vi "Main Tclk.vi"() -> ()   [LabVIEW 2018] (continued)
            n969 = property on="AF Steps" class="DigNum (strict)"("DisabledEnum"=w5460) -> ()  [unwired: 2 in, 2 out]
            n970 = property on="AS Steps" class="DigNum (strict)"("DisabledEnum"=w5460) -> ()  [unwired: 2 in, 2 out]
            n971 = property on="AA Steps" class="DigNum (strict)"("DisabledEnum"=w5460) -> ()  [unwired: 2 in, 2 out]
            n972 = property on="Beam blanked" class="Bool (strict)"("DisabledEnum"=w5460) -> ()  [unwired: 2 in, 2 out]
            n973 = property on="Spot" class="Bool (strict)"("DisabledEnum"=w5460) -> ()  [unwired: 2 in, 2 out]
            n974 = property on="Mill Stop" class="Bool (strict)"("DisabledEnum"=w5460) -> ()  [unwired: 2 in, 2 out]
            n975 = property on="ROI" class="Bool (strict)"("DisabledEnum"=w5460) -> ()  [unwired: 2 in, 2 out]
            n976 = property on="FIB Profile" class="Bool (strict)"("DisabledEnum"=w5460) -> ()  [unwired: 2 in, 2 out]
            n977 = property on="FIB FOV (um)" class="DigNum (strict)"("DisabledEnum"=w5460) -> ()  [unwired: 2 in, 2 out]
            n978 = property on="X center (um)" class="DigNum (strict)"("DisabledEnum"=w5460) -> ()  [unwired: 2 in, 2 out]
            n979 = property on="Z center (um)" class="DigNum (strict)"("DisabledEnum"=w5460) -> ()  [unwired: 2 in, 2 out]
            n980 = property on="X size (um)" class="DigNum (strict)"("DisabledEnum"=w5460) -> ()  [unwired: 2 in, 2 out]
            n981 = property on="Z size (um)" class="DigNum (strict)"("DisabledEnum"=w5460) -> ()  [unwired: 2 in, 2 out]
            n982 = property on="X resolution" class="DigNum (strict)"("DisabledEnum"=w5460) -> ()  [unwired: 2 in, 2 out]
            n983 = property on="Z resolution" class="DigNum (strict)"("DisabledEnum"=w5460) -> ()  [unwired: 2 in, 2 out]
            n984 = property on="Z-step (nm)" class="DigNum (strict)"("DisabledEnum"=w5460) -> ()  [unwired: 2 in, 2 out]
            n985 = property on="Start Current DataLog" class="Bool (strict)"("DisabledEnum"=w5460) -> ()  [unwired: 2 in, 2 out]
            n986 = local read "Machine Type"() -> (w5461:u8)
            n987 = local read "Unfreeze"() -> (w5468:bool)
            n988 = case shown="2" w5461 {
              frame 0, Default {
              }
              frame 2 {
                n989 = local read "Api"() -> (w5476:refnum<k7>)
                n990 = call "SmartSEM Remote API set float.vi"("vValue"=sgl 0.0, "lpszParam"="DP_PANEL_DISABLE", "Api"=w5476) -> ("Api out"=w5472:refnum<k7>)  [unwired: 7 in, 1 out]
                n991 = call "SmartSEM Remote API set float.vi"("vValue"=sgl 0.0, "lpszParam"="DP_JOYSTICK_DISABLE", "Api"=w5472) -> ()  [unwired: 7 in, 2 out]
              }
            }
            n992 = case shown="False" w5468 {
              tunnel: w5460 -> [w5477 _]
              frame False {
                n993 = property on="Pre image" class="Bool (strict)"("DisabledEnum"=w5477) -> ()  [unwired: 2 in, 2 out]
                n994 = property on="Post image" class="Bool (strict)"("DisabledEnum"=w5477) -> ()  [unwired: 2 in, 2 out]
                n995 = property on="Mill" class="Bool (strict)"("DisabledEnum"=w5477) -> ()  [unwired: 2 in, 2 out]
                n996 = property on="Mill Manual Pause" class="Bool (strict)"("DisabledEnum"=w5477) -> ()  [unwired: 2 in, 2 out]
              }
              frame True {
              }
            }
            n997 = property on="Pause for reheat" class="Bool (strict)"("DisabledEnum"=T44."Disabled and Grayed Out" ("Disabled")) -> ()  [unwired: 2 in, 2 out]
          }
          frame True {
            n998 = stacked-sequence {
              tunnel: [_ _ _ _ _ _ _ w5766 _ _ _ _ _ _ _ _ _ _ _ _ _ _ _ _ _ _ _ _ _ _ _ _ _ _ _ _ _ _ _ _ _ _ _] -> w5478
              frame #0 {
                w5479 = T44."Disabled and Grayed Out" ("Disabled")
                n999 = local read "FIB HW Config"() -> (w5490:T23)
                n1000 = local read "FIB HW Config"() -> (w5493:T23)
                n1001 = local read "Api"() -> (w5480:refnum<k7>)
                n1002 = Unbundle By Name(w5490) -> ("Beam blank"=w5491:tag)
                n1003 = Unbundle By Name(w5493) -> ("FIB Ext Scan"=w5494:tag)
                n1004 = local read "Milling para"() -> (w5486:T35)
                n1005 = property on="Pause for reheat" class="Bool (strict)"("DisabledEnum"=T44."Enabled" ("Disabled")) -> ()  [unwired: 2 in, 2 out]
                n1006 = property on="Scan x1" class="Bool (strict)"("DisabledEnum"=w5479) -> ()  [unwired: 2 in, 2 out]
                n1007 = property on="Mill start from Last" class="Bool (strict)"("DisabledEnum"=w5479) -> ()  [unwired: 2 in, 2 out]
                n1008 = property on="Scan xn" class="Bool (strict)"("DisabledEnum"=w5479) -> ()  [unwired: 2 in, 2 out]
                n1009 = property on="FIB Imaging" class="Bool (strict)"("DisabledEnum"=w5479) -> ()  [unwired: 2 in, 2 out]
                n1010 = property on="FIB time lapse" class="Bool (strict)"("DisabledEnum"=w5479) -> ()  [unwired: 2 in, 2 out]
                n1011 = property on="Reset" class="Bool (strict)"("DisabledEnum"=w5479) -> ()  [unwired: 2 in, 2 out]
                n1012 = property on="Pre image" class="Bool (strict)"("DisabledEnum"=w5479) -> ()  [unwired: 2 in, 2 out]
                n1013 = property on="Post image" class="Bool (strict)"("DisabledEnum"=w5479) -> ()  [unwired: 2 in, 2 out]
                n1014 = call "FIB ext scan.vi"("Ext on"=TRUE, "FIB Ext Scan"=w5494) -> ()  [unwired: 9 in, 1 out]
                n1015 = call "FIB beam blank.vi"("Api"=w5480, "Beam blanked"=TRUE, "lines"=w5491) -> ()  [unwired: 2 in, 1 out]
                n1016 = Unbundle By Name(w5486) -> ("Mill start from Last"=w5485:bool)
                n1017 = property on="Beam blanked" class="Bool (strict)"("DisabledEnum"=w5479) -> ()  [unwired: 2 in, 2 out]
                n1018 = property on="FIB Profile" class="Bool (strict)"("DisabledEnum"=w5479) -> ()  [unwired: 2 in, 2 out]
                n1019 = property on="Start Current DataLog" class="Bool (strict)"("DisabledEnum"=w5479) -> ()  [unwired: 2 in, 2 out]
                n1020 = property on="Spot" class="Bool (strict)"("DisabledEnum"=w5479) -> ()  [unwired: 2 in, 2 out]
                n1021 = property on="Mill Stop" class="Bool (strict)"("DisabledEnum"=w5479) -> ()  [unwired: 2 in, 2 out]
                n1022 = property on="ROI" class="Bool (strict)"("DisabledEnum"=w5479) -> ()  [unwired: 2 in, 2 out]
                n1023 = property on="Mill" class="Bool (strict)"("DisabledEnum"=w5479) -> ()  [unwired: 2 in, 2 out]
                n1024 = local read "FIB slice #"() -> (w5489:u32)
                n1025 = shared-variable "My Computer\\Zeiss Library.lvlib\\Milling cont. from Last"(w5485) -> ()  [unwired: 1 in, 1 out]
                n1026 = local write "SW error warning armed"(TRUE ("SW error warning armed")) -> ()
                n1027 = local write "Start Current DataLog"(FALSE ("Start Current DataLog")) -> ()
                n1028 = property on="FIB FOV (um)" class="DigNum (strict)"("DisabledEnum"=w5479) -> ()  [unwired: 2 in, 2 out]
                n1029 = property on="X center (um)" class="DigNum (strict)"("DisabledEnum"=w5479) -> ()  [unwired: 2 in, 2 out]
                n1030 = property on="X resolution" class="DigNum (strict)"("DisabledEnum"=w5479) -> ()  [unwired: 2 in, 2 out]
                n1031 = property on="Z resolution" class="DigNum (strict)"("DisabledEnum"=w5479) -> ()  [unwired: 2 in, 2 out]
                n1032 = property on="Z-step (nm)" class="DigNum (strict)"("DisabledEnum"=w5479) -> ()  [unwired: 2 in, 2 out]
                n1033 = property on="Z center (um)" class="DigNum (strict)"("DisabledEnum"=w5479) -> ()  [unwired: 2 in, 2 out]
                n1034 = property on="X size (um)" class="DigNum (strict)"("DisabledEnum"=w5479) -> ()  [unwired: 2 in, 2 out]
                n1035 = property on="Z size (um)" class="DigNum (strict)"("DisabledEnum"=w5479) -> ()  [unwired: 2 in, 2 out]
                n1036 = Equal To 0?(x=w5489) -> (x = 0?=w5488:bool)
                n1037 = And(x=w5488, y=w5485) -> (x .and. y?=w5487:bool)
                n1038 = case shown="True" w5487 {
                  frame False {
                  }
                  frame True {
                    n1039 = stacked-sequence {
                      frame #0 {
                        w5495 = TRUE ("Temperature warning armed")
                        n1040 = local read "Last FIB recipe"() -> (w5496:path)
                        n1041 = local write "Temperature warning armed"(w5495) -> ()
                        n1042 = local write "SW error warning armed"(w5495) -> ()
                        n1043 = local write "Focus index warning armed"(w5495) -> ()
                        n1044 = local write "Re-engage warning armed"(w5495) -> ()
                        n1045 = shared-variable ".\\Zeiss Library.lvlib\\FIB PID reset"(w5495) -> ()  [unwired: 1 in, 1 out]
                        n1046 = local write "Read recipe path"(w5496) -> ()
                      }
                      frame #1 {
                        n1047 = local write "Load recipe"(TRUE ("Load recipe")) -> ()
                      }
                      frame #2 {
                        n1048 = while {
                          stop <- w5498 stop-if-true
                          n1049 = local read "Load recipe"() -> (w5502:bool)
                          n1050 = Wait Until Next ms Multiple(millisecond multiple=u32 100) -> ()  [unwired: 1 out]
                          n1051 = local read "FIB"() -> (w5503:bool)
                          n1052 = local read "Stop"() -> (w5499:bool)
                          n1053 = Not(x=w5502) -> (.not. x?=w5501:bool)
                          n1054 = Not(x=w5503) -> (.not. x?=w5500:bool)
                          n1055 = Compound Arithmetic op=OR(w5501, w5500, w5499) -> (w5498:bool)
                        }
                      }
                      frame #3 {
                        n1056 = local read "Last milling snapshot"() -> (w5527:path)
                        n1057 = local read "Milling para"() -> (w5530:T35)
                        n1058 = local read "SEM Options"() -> (w5510:T27)
                        n1059 = local read "Last FIB image"() -> (w5539:path)
                        n1060 = local read "Last Det A Low Mag"() -> (w5537:path)
                        n1061 = local read "Last Det B Low Mag"() -> (w5538:path)
                        n1062 = shared-variable "My Computer\\Zeiss Library.lvlib\\Milling cont. from Last"(TRUE ("Milling cont. from Last")) -> ()  [unwired: 1 in, 1 out]
                        n1063 = local write "Initial Options"(w5510) -> ()
                        n1064 = local write "Reset Focus"(FALSE ("Reset Focus")) -> ()
                        n1065 = Bundle By Name(cluster=w5530, "Z offset (um)"=sgl 0.0 ("Y offset (um)")) -> (w5529:T35)
                        n1066 = call-poly <vilib>:"Read From XML File.vi"("XML File Path"=w5527) -> ("XML Elements"=w5526:string)  [unwired: 8 in, 2 out]
                        n1067 = File/Directory Info(path=w5539) -> (path out=w5541:path, error out=w5542:errorcluster)  [unwired: 1 in, 5 out]
                        n1068 = File/Directory Info(path=w5537) -> (path out=w5532:path, error out=w5531:errorcluster)  [unwired: 1 in, 5 out]
                        n1069 = File/Directory Info(path=w5538) -> (path out=w5535:path, error out=w5536:errorcluster)  [unwired: 1 in, 5 out]
                        n1070 = Unbundle By Name(w5542) -> ("status"=w5540:bool)
                        n1071 = Unbundle By Name(w5531) -> ("status"=w5533:bool)
                        n1072 = Unbundle By Name(w5536) -> ("status"=w5534:bool)
                        n1073 = local write "Milling para"(w5529) -> ()
                        n1074 = Unflatten From XML(xml string=w5526, type=T47 {"Timestamp"=timestamp(0 s since 1904-01-01), "Double"=0.0, "FIB slice #"=0, "Reheat"=FALSE, "Double 2"=0.0, "Double 3"=0.0, "Double 4"=0.0} ("output cluster")) -> (value=w5525:T47)  [unwired: 1 in, 1 out]
                        n1075 = case shown="False" w5540 {
                          tunnel: w5541 -> [w5558 _]
                          frame False {
                            n1076 = call <vilib>:"Read PNG File.vi"("path to PNG file"=w5558) -> ("image data"=w5559:T55)  [unwired: 8 in, 2 out]
                            n1077 = call <vilib>:"Unflatten Pixmap.vi"("image data"=w5559) -> ("8-bit pixmap"=w5557:u8[][])  [unwired: 4 in, 6 out]
                            n1078 = To Word Integer(number=w5557) -> (16bit integer=w5556:i16[][])
                            n1079 = local write "FIB Image"(w5556) -> ()
                            n1080 = shared-variable ".\\Zeiss Library.lvlib\\FIB Img"(w5556) -> ()  [unwired: 1 in, 1 out]
                          }
                          frame True {
                          }
                        }
                        n1081 = case shown="False" w5533 {
                          tunnel: w5532 -> [w5554 _]
                          frame False {
                            n1082 = call <vilib>:"Read PNG File.vi"("path to PNG file"=w5554) -> ("image data"=w5555:T55)  [unwired: 8 in, 2 out]
                            n1083 = call <vilib>:"Unflatten Pixmap.vi"("image data"=w5555) -> ("8-bit pixmap"=w5552:u8[][])  [unwired: 4 in, 6 out]
                            n1084 = To Word Integer(number=w5552) -> (16bit integer=w5553:i16[][])
                            n1085 = local write "Detector A Low Mag"(w5553) -> ()
                          }
                          frame True {
                          }
                        }
                        n1086 = case shown="False" w5534 {
                          tunnel: w5535 -> [w5550 _]
                          frame False {
                            n1087 = call <vilib>:"Read PNG File.vi"("path to PNG file"=w5550) -> ("image data"=w5551:T55)  [unwired: 8 in, 2 out]
                            n1088 = call <vilib>:"Unflatten Pixmap.vi"("image data"=w5551) -> ("8-bit pixmap"=w5549:u8[][])  [unwired: 4 in, 6 out]
                            n1089 = To Word Integer(number=w5549) -> (16bit integer=w5548:i16[][])
                            n1090 = local write "Detector B Low Mag"(w5548) -> ()
                          }
                          frame True {
                          }
                        }
                        n1091 = Unbundle(w5525) -> ("Timestamp"=w5522:timestamp, "Double"=w5524:sgl, "FIB slice #"=w5523:u32, "Reheat"=w5520:bool, "Double 2"=w5519:sgl, "Double 4"=w5506:sgl)  [unwired: 1 out]
                        "Reheat from last" <- w5520
                        n1092 = local read "Hardware Configuration"() -> (w5507:T25)
                        n1093 = Bundle By Name(cluster=w5507, "SEM Max FOV (um)"=w5506) -> (w5505:T25)
                        n1094 = Increment(x=w5523) -> (x+1=w5511:u32)
                        n1095 = case shown="True" w5520 {
                          tunnel: w5522 -> [_ w5547]
                          tunnel: w5519 -> [_ w5546]
                          frame False {
                            n1096 = local write "Pause for reheat"(FALSE ("Reheat")) -> ()
                            n1097 = property on="Pause for reheat" class="Bool (strict)"("DisabledEnum"=T44."Enabled" ("Disabled")) -> ()  [unwired: 2 in, 2 out]
                          }
                          frame True {
                            n1098 = local write "Pre-reheat time"(w5547) -> ()
                            n1099 = local write "Pre-reheat FI"(w5546) -> ()
                            n1100 = property on="Pause for reheat" class="Bool (strict)"("DisabledEnum"=T44."Disabled and Grayed Out" ("Disabled")) -> ()  [unwired: 2 in, 2 out]
                          }
                        }
                        n1101 = shared-variable ".\\Zeiss Library.lvlib\\Milling Z Voltage Last"(w5524) -> ()  [unwired: 1 in, 1 out]
                        n1102 = local write "FIB slice #"(w5511) -> ()
                        n1103 = local read "Email Alert Recipients"() -> (w5515:string[])
                        n1104 = local write "Hardware Configuration"(w5505) -> ()
                        n1105 = local read "Email recipents file"() -> (w5512:path)
                        n1106 = Open/Create/Replace File(file path (use dialog)=w5512, operation (0:open)=T49."replace or create") -> (refnum out=w5513:refnum<file>, error out=w5514:errorcluster)  [unwired: 4 in, 1 out]
                        n1107 = Write to Text File(file (use dialog)=w5513, text=w5515, error in=w5514) -> (refnum out=w5516:refnum<file>, error out=w5517:errorcluster)  [unwired: 1 in, 1 out]
                        n1108 = Close File(refnum=w5516, error in=w5517) -> ()  [unwired: 2 out]
                      }
                      frame #4 {
                        n1109 = local read "Reheat from last"() -> (w5560:bool)
                        n1110 = case shown="True" w5560 {
                          frame False {
                          }
                          frame True {
                            n1111 = local read "SEM Scan Parameters"() -> (w5565:T26)
                            n1112 = Unbundle By Name(w5565) -> ("X center (um)"=w5564:sgl, "Y center (um)"=w5563:sgl, "Y stig"=w5562:sgl[][])
                            n1113 = local write "Pre-reheat X center (um)"(w5564) -> ()
                            n1114 = local write "Pre-reheat Y center (um)"(w5563) -> ()
                            n1115 = local write "Pre-reheat Y stig"(w5562) -> ()
                            n1116 = local write "Status Tabs"(T11."Re-engage" ("Status Tabs")) -> ()
                          }
                        }
                      }
                    }
                  }
                }
              }
              frame #1 {
                n1117 = local read "Machine Type"() -> (w5582:u8)
                n1118 = local read "Milling para"() -> (w5580:T35)
                n1119 = Unbundle By Name(w5580) -> ("Lines auto pause"=w5579:u16)
                n1120 = case shown="2" w5582 {
                  tunnel: [w5591 w5599 w5603] -> w5583
                  frame 0, Default {
                    n1121 = for {
                      N: 10 -> [_]
                      tunnel: [w5596] -> w5593 mode=indexing
                      n1122 = shared-variable ".\\Zeiss Library.lvlib\\Logs"() -> (w5598:sgl[])  [unwired: 1 in, 1 out]
                      n1123 = Wait Until Next ms Multiple(millisecond multiple=u32 10) -> ()  [unwired: 1 out]
                      n1124 = Index Array(array=w5598, index=0) -> (element=w5596:sgl)
                    }
                    n1125 = call-poly <vilib>:"Basic Averaged DC-RMS.vi"("signal in"=w5593) -> ("DC value"=w5592:dbl)  [unwired: 7 in, 3 out]
                    n1126 = To Single Precision Float(number=w5592) -> (single precision float=w5591:sgl)
                  }
                  frame 1 {
                    n1127 = local read "Faraday Cup (nA)"() -> (w5599:sgl)
                  }
                  frame 2 {
                    n1128 = local read "Api"() -> (w5602:refnum<k7>)
                    n1129 = for {
                      N: 10 -> [_]
                      tunnel: [w5608] -> w5605 mode=indexing
                      n1130 = shared-variable ".\\Zeiss Library.lvlib\\Logs"() -> (w5610:sgl[])  [unwired: 1 in, 1 out]
                      n1131 = Wait Until Next ms Multiple(millisecond multiple=u32 10) -> ()  [unwired: 1 out]
                      n1132 = Index Array(array=w5610, index=0) -> (element=w5608:sgl)
                    }
                    n1133 = call "SmartSEM Remote API set float.vi"("vValue"=sgl 1.0, "lpszParam"="DP_PANEL_DISABLE", "Api"=w5602) -> ()  [unwired: 7 in, 2 out]
                    n1134 = call-poly <vilib>:"Basic Averaged DC-RMS.vi"("signal in"=w5605) -> ("DC value"=w5604:dbl)  [unwired: 7 in, 3 out]
                    n1135 = To Single Precision Float(number=w5604) -> (single precision float=w5603:sgl)
                  }
                }
                "Faraday Cup before mill" <- w5583
                n1136 = Equal?(x=w5579, y=u16 1) -> (x = y?=w5572:bool)
                n1137 = case shown="True" w5572 {
                  tunnel: [0 w5585] -> w5571
                  frame False {
                  }
                  frame True {
                    n1138 = local read "Continued fine milling frames"() -> (w5586:i32)
                    n1139 = Increment(x=w5586) -> (x+1=w5585:i32)
                  }
                }
                n1140 = local read "EHT off"() -> (w5575:bool)
                n1141 = local read "Faraday Cup (nA)"() -> (w5577:sgl)
                n1142 = local read "SEM Options"() -> (w5581:T27)
                n1143 = Not(x=w5575) -> (.not. x?=w5574:bool)
                n1144 = Unbundle By Name(w5581) -> ("Upload"=w5567:bool)
                n1145 = Greater?(x=w5577, y=sgl 0.1) -> (0:w5573:bool)
                n1146 = shared-variable ".\\Zeiss Library.lvlib\\Faraday Cup before mill"(w5583) -> ()  [unwired: 1 in, 1 out]
                n1147 = local write "Continued fine milling frames"(w5571) -> ()
                n1148 = Greater?(x=w5571, y=5) -> (0:w5569:bool)
                n1149 = Compound Arithmetic op=AND(w5569, w5574, w5573) -> (w5568:bool)
                n1150 = Or(x=w5568, y=w5567) -> (x .or. y?=w5566:bool)
                n1151 = case shown="True" w5566 {
                  frame False {
                  }
                  frame True {
                    w5588 = TRUE ("Upload")
                    n1152 = local read "Alert Settings"() -> (w5590:T36)
                    n1153 = Bundle By Name(cluster=w5590, "3D imaging paused alarm"=w5588, "FIB emission warning"=w5588, "Specimen @ SEM alarm"=w5588, "FIB CL current alarm"=w5588, "Beam Dump 1 alarm"=w5588, "Milling Z voltage alarm"=w5588, "EHT off alarm"=w5588, "Image clipping alarm"=w5588, "Temperature alarm"=w5588, "SW error warning"=w5588, "Focus index warning"=w5588) -> (w5589:T36)
                    n1154 = local write "Coarse milling"(FALSE ("Coarse milling")) -> ()
                    n1155 = local write "Alert Settings"(w5589) -> ()
                  }
                }
              }
              frame #2 {
                w5612 = FALSE ("Rect Milling Line Paused")
                w5613 = TRUE ("Auto pause")
                n1156 = local read "Milling para"() -> (w5611:T35)
                n1157 = Bundle By Name(cluster=w5611, "Auto pause"=w5613) -> (w5614:T35)
                n1158 = shared-variable "My Computer\\Zeiss Library.lvlib\\Milling Resume"(w5613) -> ()  [unwired: 1 in, 1 out]
                n1159 = shared-variable "My Computer\\Zeiss Library.lvlib\\Milling Line Paused"(w5612) -> ()  [unwired: 1 in, 1 out]
                n1160 = local write "Mill Stop"(w5612) -> ()
                n1161 = local write "Milling para"(w5614) -> ()
              }
              frame #3 {
                n1162 = local read "FIB slice #"() -> (w5616:u32)
                n1163 = Equal To 0?(x=w5616) -> (x = 0?=w5615:bool)
                n1164 = case shown="True" w5615 {
                  frame False {
                  }
                  frame True {
                    n1165 = stacked-sequence {
                      frame #0 {
                        w5630 = 0.0
                        w5641 = TRUE ("Temperature warning armed")
                        w5619 = u32[] [] ("Log time array")
                        w5617 = sgl[] []
                        n1166 = local write "SW error warning armed"(w5641) -> ()
                        n1167 = local write "Focus index warning armed"(w5641) -> ()
                        n1168 = local write "Temperature warning armed"(w5641) -> ()
                        n1169 = local write "Re-engage warning armed"(w5641) -> ()
                        n1170 = shared-variable ".\\Zeiss Library.lvlib\\FIB PID reset"(w5641) -> ()  [unwired: 1 in, 1 out]
                        n1171 = Get Date/Time In Seconds() -> (seconds since 1Jan1904=w5640:timestamp)
                        n1172 = To Double Precision Float(number=w5640) -> (double precision float=w5635:dbl)
                        n1173 = Bundle(w5630, w5630) -> (w5629:cluster{dbl, dbl})  [unwired: 1 in]
                        n1174 = Add(x=w5635, y=86400.0 ("X Scale.Range:Maximum")) -> (x+y=w5637:dbl)
                        n1175 = Initialize Array(w5629, 0) -> (w5632:cluster{dbl, dbl}[])
                        n1176 = Add(x=w5635, y=0.0 ("X Scale.Range:Minimum")) -> (x+y=w5633:dbl)
                        n1177 = local read "SEM Scan Parameters"() -> (w5623:T26)
                        n1178 = property on="FIB HV DataLog" class="WFChart (strict)"("History Data"=w5632, "XScale.Offset"=w5635, "XScale.Minimum"=w5633, "XScale.Maximum"=w5637, "XScale.Increment"=14400.0 ("X Scale.Range:Increment"), "XScale.MinorInc"=3600.0 ("X Scale.Range:Minor Increment")) -> ()  [unwired: 2 in, 2 out]
                        n1179 = Unbundle By Name(w5623) -> ("Y tiles"=w5622:u8, "X tiles"=w5621:u8)
                        n1180 = Initialize Array(FALSE ("run minimized? (F)"), w5622, w5621) -> (w5624:bool[][])
                        n1181 = local read "3D FIB-SEM Files"() -> (w5627:path)
                        n1182 = local write "AF Success tiled"(w5624) -> ()
                        n1183 = local write "ASX Success tiled"(w5624) -> ()
                        n1184 = local write "ASY Success tiled"(w5624) -> ()
                        n1185 = local write "AAX Success tiled"(w5624) -> ()
                        n1186 = local write "AAY Success tiled"(w5624) -> ()
                        n1187 = local write "Auto re-engage"(FALSE ("Auto re-engage")) -> ()
                        n1188 = call <vilib>:"System Exec.vi"("run minimized? (F)"=TRUE, "working directory"=w5627, "command line"="cmd /c del Primary_grid*.png pre*.png post*.png") -> ()  [unwired: 5 in, 4 out]
                        "Temp array" <- w5617
                        "Faraday Cup array" <- w5617
                        "Specimen I array" <- w5617
                        "Beam Dump 1 array" <- w5617
                        "Log time array" <- w5619
                        "Delta X array" <- w5617
                        "Delta Y array" <- w5617
                        "Delta image array" <- w5617
                        "Focus index array" <- w5617
                        "Delta X sum array" <- w5617
                        "Delta Y sum array" <- w5617
                        "SEM Specimen I array" <- w5617
                        "Milling Z voltage array" <- w5617
                        "Delta Z array" <- w5617
                        "Beam Dump 2 array" <- w5617
                        "Milling I array" <- w5617
                        "Temp low limit array" <- w5617
                        "Temp high limit array" <- w5617
                        "SEM Specimen I low limit array" <- w5617
                        "SEM Specimen I high limit array" <- w5617
                        "FI low limit array" <- w5617
                        "Specimen I low limit array" <- w5617
                        "Specimen I high limit array" <- w5617
                        "Faraday Cup low limit array" <- w5617
                        "Faraday Cup high limit array" <- w5617
                        "Cycle time array" <- w5619
                        "Cycle time est offset array" <- i16[] [] ("Log time array")
                        "BD1 low limit array" <- w5617
                        "BD1 high limit array" <- w5617
                        "BD2 low limit array" <- w5617
                        "BD2 high limit array" <- w5617
                        "Milling I low limit array" <- w5617
                        "Milling I high limit array" <- w5617
                        "FI low warning limit array" <- w5617
                        "FI high warning limit array" <- w5617
                        "FI low stop limit array" <- w5617
                        "FI high stop limit array" <- w5617
                        "Delta X stop limit array" <- w5617
                        "Delta Y stop limit array" <- w5617
                        "FI array for stop limit" <- w5617
                        "Delta X array for stop limit" <- w5617
                        "Delta Y array for stop limit" <- w5617
                      }
                      frame #1 {
                        n1189 = local read "SEM Scan Parameters"() -> (w5668:T26)
                        n1190 = Unbundle By Name(w5668) -> ("WD (mm)"=w5667:sgl[][], "X stig"=w5664:sgl[][], "Y stig"=w5661:sgl[][], "X aln"=w5660:sgl[][], "Y aln"=w5658:sgl[][], "dX (um)"=w5656:sgl[], "dY (um)"=w5651:sgl[], "Y tiles"=w5654:u8, "X tiles"=w5652:u8)
                        n1191 = local read "WD Stig Aln tile offsets"() -> (w5670:T3)
                        n1192 = Build Array(w5654, w5652) -> (w5657:u8[])
                        n1193 = Array Size(array=w5667) -> (size(s)=w5666:i32[])
                        n1194 = Array Size(array=w5664) -> (size(s)=w5665:i32[])
                        n1195 = Array Size(array=w5661) -> (size(s)=w5662:i32[])
                        n1196 = Array Size(array=w5660) -> (size(s)=w5663:i32[])
                        n1197 = Array Size(array=w5658) -> (size(s)=w5659:i32[])
                        n1198 = Array Size(array=w5656) -> (size(s)=w5655:i32)
                        n1199 = Array Size(array=w5651) -> (size(s)=w5653:i32)
                        n1200 = Equal?(x=w5666, y=w5657) -> (x = y?=w5649:bool[])
                        n1201 = Equal?(x=w5665, y=w5657) -> (x = y?=w5648:bool[])
                        n1202 = Equal?(x=w5662, y=w5657) -> (x = y?=w5646:bool[])
                        n1203 = Equal?(x=w5663, y=w5657) -> (x = y?=w5645:bool[])
                        n1204 = Equal?(x=w5659, y=w5657) -> (x = y?=w5644:bool[])
                        n1205 = Equal?(x=w5655, y=w5654) -> (x = y?=w5643:bool)
                        n1206 = Equal?(x=w5653, y=w5652) -> (x = y?=w5642:bool)
                        n1207 = Build Array (concatenate)(w5649, w5648, w5646, w5645, w5644, w5643, w5642) -> (w5647:bool[])
                        n1208 = And Array Elements(Boolean array=w5647) -> (logical AND=w5650:bool)
                        n1209 = case shown="True" w5650 {
                          tunnel: [w5671 w5699] -> w5669
                          tunnel: w5668 -> [w5673 w5693]
                          tunnel: w5670 -> [w5672 w5680]
                          frame False {
                            w5675 = sgl 0.0 ("element")
                            n1210 = Unbundle By Name(w5673) -> ("Y tiles"=w5677:u8, "X tiles"=w5679:u8)
                            n1211 = Initialize Array(w5675, w5677, w5679) -> (w5678:sgl[][])
                            n1212 = Initialize Array(w5675, w5677) -> (w5676:sgl[])
                            n1213 = Initialize Array(w5675, w5679) -> (w5674:sgl[])
                            n1214 = Bundle By Name(cluster=w5672, "dWD"=w5678, "dX stig"=w5678, "dY stig"=w5678, "dX aln"=w5678, "dY aln"=w5678, "dX (um)"=w5676, "dY (um)"=w5674) -> (w5671:T3)
                          }
                          frame True {
                            n1215 = Unbundle By Name(w5693) -> ("WD (mm)"=w5689:sgl[][], "X stig"=w5687:sgl[][], "Y stig"=w5684:sgl[][], "X aln"=w5683:sgl[][], "Y aln"=w5681:sgl[][], "dX (um)"=w5700:sgl[], "dY (um)"=w5705:sgl[], "Y tiles"=w5692:u8, "X tiles"=w5691:u8)
                            n1216 = expression code="(x-1)/2"(w5692) -> (w5703:u8)
                            n1217 = expression code="(x-1)/2"(w5691) -> (w5706:u8)
                            n1218 = Index Array(array=w5689, index (row)=w5703, index (col)=w5706) -> (element=w5690:sgl)
                            n1219 = Index Array(array=w5687, index (row)=w5703, index (col)=w5706) -> (element=w5688:sgl)
                            n1220 = Index Array(array=w5684, index (row)=w5703, index (col)=w5706) -> (element=w5685:sgl)
                            n1221 = Index Array(array=w5683, index (row)=w5703, index (col)=w5706) -> (element=w5686:sgl)
                            n1222 = Index Array(array=w5681, index (row)=w5703, index (col)=w5706) -> (element=w5682:sgl)
                            n1223 = Index Array(array=w5700, index=w5703) -> (element=w5701:sgl)
                            n1224 = Index Array(array=w5705, index=w5706) -> (element=w5704:sgl)
                            n1225 = Subtract(x=w5689, y=w5690) -> (x-y=w5694:sgl[][])
                            n1226 = Subtract(x=w5687, y=w5688) -> (x-y=w5695:sgl[][])
                            n1227 = Subtract(x=w5684, y=w5685) -> (x-y=w5696:sgl[][])
                            n1228 = Subtract(x=w5683, y=w5686) -> (x-y=w5697:sgl[][])
                            n1229 = Subtract(x=w5681, y=w5682) -> (x-y=w5698:sgl[][])
                            n1230 = Subtract(x=w5700, y=w5701) -> (x-y=w5702:sgl[])
                            n1231 = Subtract(x=w5705, y=w5704) -> (x-y=w5707:sgl[])
                            n1232 = Bundle By Name(cluster=w5680, "dWD"=w5694, "dX stig"=w5695, "dY stig"=w5696, "dX aln"=w5697, "dY aln"=w5698, "dX (um)"=w5702, "dY (um)"=w5707) -> (w5699:T3)
                          }
                        }
                        n1233 = local write "WD Stig Aln tile offsets"(w5669) -> ()
                      }
                    }
                  }
                }
              }
              frame #4 {
                n1234 = Unbundle By Name("Low Mag SEM") -> ("Low mag scan"=w5710:bool)
                n1235 = Unbundle By Name("Mid Mag SEM") -> ("Mid mag scan"=w5711:bool)
                n1236 = case shown="True" w5710 {
                  tunnel: "Low Mag SEM" -> [_ w5734]
                  frame False {
                  }
                  frame True {
                    w5730 = sgl[] [0.0] ("dX (um)")
                    w5731 = u8 1 ("X tiles")
                    w5735 = 0.0 ("X center")
                    n1237 = Unbundle By Name(w5734) -> ("Low mag scan FOV (micron)"=w5732:dbl, "Low mag scan rate (Hz)"=w5744:u32)
                    n1238 = local read "SEM Scan Parameters"() -> (w5737:T26)
                    n1239 = Unbundle By Name(w5737) -> ("Scan rate (Hz)"=w5739:u32, "Oversampling"=w5738:u32)
                    n1240 = expression code="x*1000"(w5732) -> (w5745:dbl)
                    n1241 = Multiply(x=w5739, y=w5738) -> (x*y=w5740:u32)
                    n1242 = Divide(x=w5740, y=w5744) -> (x/y=w5741:dbl)
                    n1243 = Divide(x=w5745, y=u32 512 ("X resolution")) -> (x/y=w5743:dbl)
                    n1244 = Bundle By Name(cluster=w5737, "X size (um)"=w5732, "Y size (um)"=w5732, "X center (um)"=w5735, "Y center (um)"=w5735, "X size (V)"=20.0, "Scan rate (Hz)"=w5744, "Oversampling"=w5741, "X tiles"=w5731, "Y tiles"=w5731, "Frames"=w5731, "dX (um)"=w5730, "dY (um)"=w5730, "Pixel size (nm)"=w5743) -> (→"SEM Low Mag Scan Parameters":T26)
                  }
                }
                n1245 = case shown="True" w5711 {
                  tunnel: "Mid Mag SEM" -> [_ w5718]
                  frame False {
                  }
                  frame True {
                    w5712 = sgl[] [0.0] ("dX (um)")
                    w5713 = u8 1 ("X tiles")
                    n1246 = local read "SEM Scan Parameters"() -> (w5719:T26)
                    n1247 = Unbundle By Name(w5718) -> ("X size (um)"=w5725:sgl, "Y size (um)"=w5726:sgl, "X center (um)"=w5727:dbl, "Y center (um)"=w5728:dbl, "Mid mag scan rate (Hz)"=w5724:u32, "Pixel size (nm)"=w5729:sgl)
                    n1248 = local read "SEM Mid Mag Scan Parameters"() -> (w5716:T5)
                    n1249 = Unbundle By Name(w5719) -> ("Scan rate (Hz)"=w5721:u32, "Oversampling"=w5720:u32)
                    n1250 = Unbundle By Name(w5716) -> ("X size (V)"=w5715:dbl)
                    n1251 = Multiply(x=w5721, y=w5720) -> (x*y=w5722:u32)
                    n1252 = Divide(x=w5722, y=w5724) -> (x/y=w5723:dbl)
                    n1253 = Bundle By Name(cluster=w5719, "X size (um)"=w5725, "Y size (um)"=w5726, "X center (um)"=w5727, "Y center (um)"=w5728, "Oversampling auto"=TRUE ("X size auto"), "Scan rate (Hz)"=w5724, "Oversampling"=w5723, "Pixel size (nm)"=w5729, "X size (V)"=w5715, "X tiles"=w5713, "Y tiles"=w5713, "Frames"=w5713, "dX (um)"=w5712, "dY (um)"=w5712) -> (→"SEM Mid Mag Scan Parameters":T26)
                  }
                }
              }
              frame #5 {
                w5746 = TRUE ("Mill")
                n1254 = local write "Mill"(w5746) -> ()
                n1255 = local write "Run once"(w5746) -> ()
                n1256 = Wait (ms)(milliseconds to wait=u32 200) -> ()  [unwired: 1 out]
              }
              frame #6 {
                n1257 = shared-variable ".\\Zeiss Library.lvlib\\Milling Z Voltage"() -> (w5749:sgl)  [unwired: 1 in, 1 out]
                n1258 = local read "FIB Options"() -> (w5758:T33)
                n1259 = local read "FIB Scan Parameters"() -> (w5756:T32)
                n1260 = local read "Milling para"() -> (w5755:T35)
                n1261 = Unbundle By Name(w5758) -> ("Flip z"=w5763:bool)
                n1262 = Unbundle By Name(w5755) -> ("FIB FOV (um)"=w5762:sgl)
                n1263 = Unbundle By Name(w5755) -> ("X size (um)"=w5753:sgl, "Line milling time (s)"=w5751:sgl, "Lines auto pause"=w5750:u16)
                n1264 = Unbundle By Name(w5756) -> ("Z size (V)"=w5757:dbl)
                n1265 = Negate(x=w5749) -> (-x=w5759:sgl)
                n1266 = Select(t=w5759, s=w5763, f=w5749) -> (s? t:f=w5760:sgl)
                n1267 = Divide(x=w5760, y=w5757) -> (x/y=w5761:dbl)
                n1268 = Multiply(x=w5761, y=w5762) -> (x*y=w5748:dbl)
                n1269 = call "Milling parameter to trapezoidal shape.vi"("Y location (um)"=w5748, "Milling para"=w5755) -> ("X size (um) @ Y"=w5754:dbl)  [unwired: 5 in, 4 out]
                n1270 = Divide(x=w5754, y=w5753) -> (x/y=w5752:dbl)
                n1271 = Compound Arithmetic op=MULTIPLY(w5752, w5751, w5750) -> (w5764:dbl)
                n1272 = local write "Milling time (s)"(w5764) -> ()
              }
              frame #7 {
                n1273 = while {
                  tunnel: [w5795] -> w5766
                  tunnel: [w5789] -> w5767
                  i -> [w5771]
                  stop <- w5796 stop-if-true
                  n1274 = Get Date/Time In Seconds() -> (seconds since 1Jan1904=w5785:timestamp)
                  n1275 = local read "Re-engage time"() -> (w5779:timestamp)
                  n1276 = local read "Milling para"() -> (w5782:T35)
                  n1277 = local read "Pre-reheat FIB PID target"() -> (w5778:sgl)
                  n1278 = local read "Run once"() -> (w5776:bool)
                  n1279 = shared-variable "My Computer\\Zeiss Library.lvlib\\Milling Line Paused"() -> (w5790:bool)  [unwired: 1 in, 1 out]
                  n1280 = local read "Mill Manual Pause"() -> (w5794:bool)
                  n1281 = local read "Machine Type"() -> (w5772:u8)
                  n1282 = local read "Auto reheat running"() -> (w5770:bool)
                  n1283 = local read "Reheat Output"() -> (w5788:T21)
                  n1284 = local read "Stop"() -> (w5795:bool)
                  n1285 = Wait Until Next ms Multiple(millisecond multiple=u32 100 ("milliseconds to wait")) -> ()  [unwired: 1 out]
                  n1286 = Unbundle By Name(w5782) -> ("FIB PID on"=w5780:bool)
                  n1287 = local read "FIB"() -> (w5792:bool)
                  n1288 = Subtract(x=w5785, y=w5779) -> (x-y=w5784:dbl)
                  n1289 = Unbundle By Name(w5788) -> ("Reheat Success"=w5787:bool)
                  n1290 = Not Equal To 0?(x=w5778) -> (x != 0?=w5775:bool)
                  n1291 = Not(x=w5792) -> (.not. x?=w5789:bool)
                  n1292 = expression code="x/60"(w5784) -> (w5777:dbl)
                  n1293 = case shown="True" w5794 {
                    tunnel: T44."Disabled and Grayed Out" ("Disabled") -> [w5891 _]
                    tunnel: T44."Enabled" ("Disabled") -> [_ w5909]
                    tunnel: w5772 -> [w5890 w5908]
                    tunnel: w5771 -> [w5889 w5907]
                    tunnel: w5770 -> [_ w5906]
                    frame False {
                      n1294 = stacked-sequence {
                        tunnel: w5891 -> [_ w5896 w5897 _ _]
                        tunnel: w5890 -> [_ _ _ w5898 w5902]
                        tunnel: w5889 -> [w5893 _ _ _ _]
                        frame #0 {
                          n1295 = Equal To 0?(x=w5893) -> (x = 0?=w5892:bool)
                          n1296 = case shown="True" w5892 {
                            frame False {
                            }
                            frame True {
                              n1297 = local write "Start Current DataLog"(FALSE ("Start Current DataLog")) -> ()
                              n1298 = local write "Status message"("FIB milling ..." ("Status message")) -> ()
                            }
                          }
                        }
                        frame #1 {
                          n1299 = property on="Scan x1" class="Bool (strict)"("DisabledEnum"=w5896) -> ()  [unwired: 2 in, 2 out]
                          n1300 = property on="Scan xn" class="Bool (strict)"("DisabledEnum"=w5896) -> ()  [unwired: 2 in, 2 out]
                          n1301 = property on="Pre image" class="Bool (strict)"("DisabledEnum"=w5896) -> ()  [unwired: 2 in, 2 out]
                          n1302 = property on="Post image" class="Bool (strict)"("DisabledEnum"=w5896) -> ()  [unwired: 2 in, 2 out]
                          n1303 = property on="Reset" class="Bool (strict)"("DisabledEnum"=w5896) -> ()  [unwired: 2 in, 2 out]
                          n1304 = property on="Start Current DataLog" class="Bool (strict)"("DisabledEnum"=w5896) -> ()  [unwired: 2 in, 2 out]
                        }
                        frame #2 {
                          n1305 = property on="FIB Imaging" class="Bool (strict)"("DisabledEnum"=w5897) -> ()  [unwired: 2 in, 2 out]
                          n1306 = property on="FIB time lapse" class="Bool (strict)"("DisabledEnum"=w5897) -> ()  [unwired: 2 in, 2 out]
                        }
                        frame #3 {
                          n1307 = case shown="2" w5898 {
                            frame 0, Default {
                            }
                            frame 2 {
                              n1308 = local read "Api"() -> (w5901:refnum<k7>)
                              n1309 = call "SmartSEM Remote API set float.vi"("vValue"=sgl 1.0, "lpszParam"="DP_PANEL_DISABLE", "Api"=w5901) -> ()  [unwired: 7 in, 2 out]
                            }
                          }
                        }
                        frame #4 {
                          n1310 = case shown="2" w5902 {
                            frame 0, Default {
                            }
                            frame 2 {
                              n1311 = local read "Api"() -> (w5905:refnum<k7>)
                              n1312 = call "SmartSEM Remote API set float.vi"("vValue"=sgl 1.0, "lpszParam"="DP_JOYSTICK_DISABLE", "Api"=w5905) -> ()  [unwired: 7 in, 2 out]
                            }
                          }
                        }
                      }
                    }
                    frame True {
                      n1313 = stacked-sequence {
                        tunnel: w5909 -> [_ w5916 w5917 _ _ _]
                        tunnel: w5908 -> [_ _ _ w5918 w5922 _]
                        tunnel: w5907 -> [w5914 _ _ _ _ _]
                        tunnel: w5906 -> [w5913 _ _ _ _ _]
                        frame #0 {
                          n1314 = Equal To 0?(x=w5914) -> (x = 0?=w5912:bool)
                          n1315 = Not(x=w5913) -> (.not. x?=w5911:bool)
                          n1316 = Compound Arithmetic op=AND(w5912, w5911) -> (w5910:bool)
                          n1317 = case shown="True" w5910 {
                            frame False {
                            }
                            frame True {
                              n1318 = local write "Status message"("Milling paused" ("Status message")) -> ()
                            }
                          }
                        }
                        frame #1 {
                          n1319 = property on="Scan x1" class="Bool (strict)"("DisabledEnum"=w5916) -> ()  [unwired: 2 in, 2 out]
                          n1320 = property on="Scan xn" class="Bool (strict)"("DisabledEnum"=w5916) -> ()  [unwired: 2 in, 2 out]
                          n1321 = property on="Pre image" class="Bool (strict)"("DisabledEnum"=w5916) -> ()  [unwired: 2 in, 2 out]
                          n1322 = property on="Post image" class="Bool (strict)"("DisabledEnum"=w5916) -> ()  [unwired: 2 in, 2 out]
                          n1323 = property on="Reset" class="Bool (strict)"("DisabledEnum"=w5916) -> ()  [unwired: 2 in, 2 out]
                          n1324 = property on="Start Current DataLog" class="Bool (strict)"("DisabledEnum"=w5916) -> ()  [unwired: 2 in, 2 out]
                        }
                        frame #2 {
                          n1325 = property on="FIB Imaging" class="Bool (strict)"("DisabledEnum"=w5917) -> ()  [unwired: 2 in, 2 out]
                          n1326 = property on="FIB time lapse" class="Bool (strict)"("DisabledEnum"=w5917) -> ()  [unwired: 2 in, 2 out]
                          n1327 = property on="Pause for reheat" class="Bool (strict)"("DisabledEnum"=w5917) -> ()  [unwired: 2 in, 2 out]
                        }
                        frame #3 {
                          n1328 = case shown="2" w5918 {
                            frame 0, Default {
                            }
                            frame 2 {
                              n1329 = local read "Api"() -> (w5921:refnum<k7>)
                              n1330 = call "SmartSEM Remote API set float.vi"("vValue"=sgl 0.0, "lpszParam"="DP_PANEL_DISABLE", "Api"=w5921) -> ()  [unwired: 7 in, 2 out]
                            }
                          }
                        }
                        frame #4 {
                          n1331 = case shown="2" w5922 {
                            frame 0, Default {
                            }
                            frame 2 {
                              n1332 = local read "Api"() -> (w5925:refnum<k7>)
                              n1333 = call "SmartSEM Remote API set float.vi"("vValue"=sgl 0.0, "lpszParam"="DP_JOYSTICK_DISABLE", "Api"=w5925) -> ()  [unwired: 7 in, 2 out]
                            }
                          }
                        }
                        frame #5 {
                          n1334 = local read "FIB HW Config"() -> (w5927:T23)
                          n1335 = local read "Api"() -> (w5926:refnum<k7>)
                          n1336 = Unbundle By Name(w5927) -> ("Beam blank"=w5928:tag)
                          n1337 = call "FIB beam blank.vi"("Api"=w5926, "Beam blanked"=TRUE, "lines"=w5928) -> ()  [unwired: 2 in, 1 out]
                        }
                      }
                    }
                  }
                  n1338 = Subtract(x="Transition time (min)", y=w5777) -> (x-y=w5773:dbl)
                  n1339 = Greater Than 0?(x=w5773) -> (x > 0?=w5774:bool)
                  n1340 = Compound Arithmetic op=AND(w5774, w5780, w5775, w5776) -> (w5781:bool)
                  n1341 = Compound Arithmetic op=AND(w5770, w5787) -> (w5786:bool)
                  n1342 = case shown="True" w5781 {
                    tunnel: w5777 -> [_ w5823]
                    tunnel: "Transition time (min)" -> [_ w5822]
                    tunnel: w5782 -> [w5805 w5812]
                    tunnel: w5778 -> [w5802 w5811]
                    tunnel: w5775 -> [w5801 _]
                    tunnel: w5773 -> [w5800 _]
                    frame False {
                      n1343 = Less Than 0?(x=w5800) -> (x < 0?=w5798:bool)
                      n1344 = local read "PID recovered"() -> (w5803:bool)
                      n1345 = Not(x=w5803) -> (.not. x?=w5799:bool)
                      n1346 = Compound Arithmetic op=AND(w5799, w5798, w5801) -> (w5804:bool)
                      n1347 = case shown="True" w5804 {
                        tunnel: w5805 -> [_ w5808]
                        tunnel: w5802 -> [_ w5807]
                        frame False {
                        }
                        frame True {
                          n1348 = Bundle By Name(cluster=w5808, "FIB PID target"=w5807) -> (w5809:T35)
                          n1349 = local write "Milling para"(w5809) -> ()
